vi "Load Custom Test Config Data.vi"(8 "Error In":errorcluster, 9 "Challenge Config Directory":path, 10 "Challenge Config":T1, 11 "Config File Handle":T2) -> (0 "Error Out":errorcluster, 1 "Challenge Config Directory":path, 2 "Challenge Config":T1, 3 "Config File Handle":T2)   [LabVIEW 2013, in "VIChallenge.lvlib"]
doc: "Load custom tests by reading from the challenge config file."
uses:
  VIChallenge.lvlib
  <vilib>/Utility/config.llb/Config Data RefNum.ctl
  Type Defs/Challenge.ctl
  <vilib>/Utility/config.llb/Read Key (Boolean).vi
  <vilib>/Utility/config.llb/NI_LVConfig.lvlib
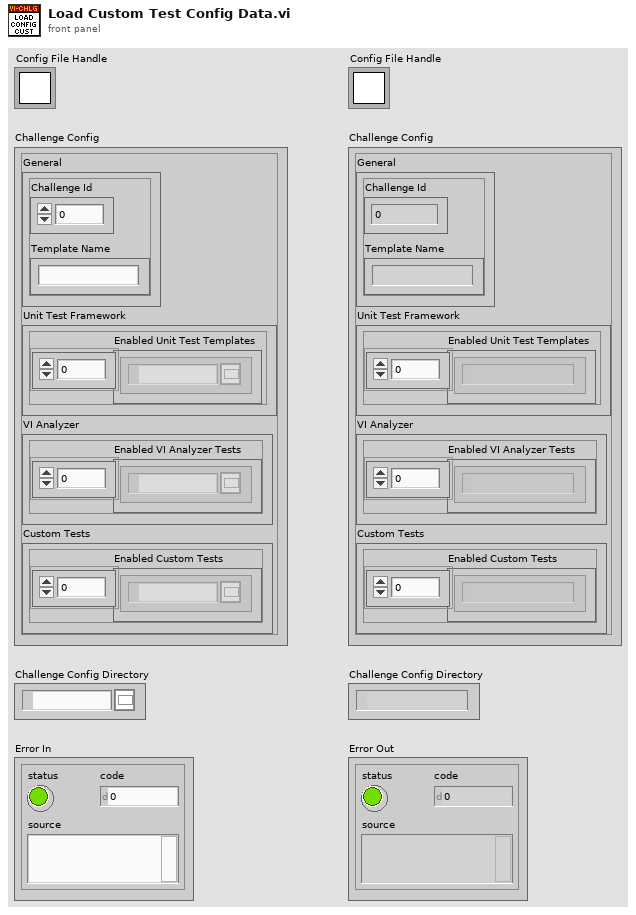
[diagram p1: front panel]
types:
  T1 = typedef "VIChallenge.lvlib/Challenge.ctl" = cluster{"General":cluster{"Challenge Id":i32, "Template Name":string}, "Unit Test Framework":cluster{"Enabled Unit Test Templates":path[]}, "VI Analyzer":cluster{"Enabled VI Analyzer Tests":path[]}, "Custom Tests":cluster{"Enabled Custom Tests":path[]}}
  T2 = typedef "NI_LVConfig.lvlib/Config Data RefNum.ctl" = refnum<k1>
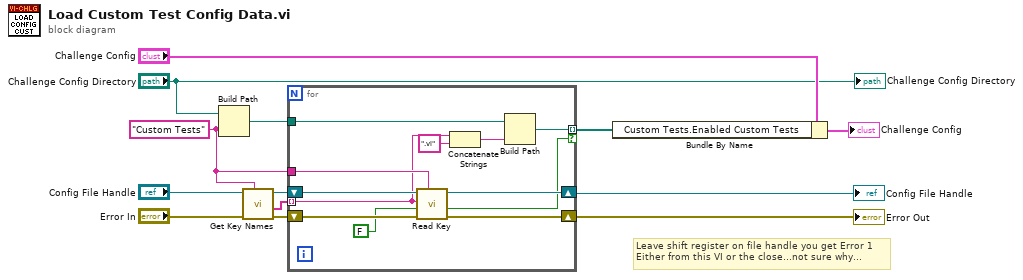
[diagram p0: block diagram]
diagram:
  w1 = "Custom Tests" ("name or relative path")
  # "Leave shift register on file handle you get Error 1\nEither from this VI or the close...not sure why..."
  n1 = Build Path(base path="Challenge Config Directory", name or relative path=w1) -> (appended path=w2:path)
  n2 = call <vilib>:"Get Key Names.vi"("section"=w1, "error in (no error)"="Error In", "refnum"="Config File Handle") -> ("error out"=w9:errorcluster, "key names"=w11:string[], "refnum out"=w10:T2)  [unwired: 5 in, 1 out]
  n3 = for {
    tunnel: w11 -> [w16] mode=indexing
    tunnel: w1 -> [w22]
    shift-right: [w20] -> w13
    shift-left: w9 -> [w25]
    tunnel: [w19] -> w4 mode=indexing if=w18
    tunnel: w2 -> [w17]
    shift-right: [w21] -> w12
    shift-left: w10 -> [w24]
    n4 = call-poly <vilib>:"Read Key.vi"("section"=w22, "error in (no error)"=w25, "default value"=FALSE, "key"=w16, "refnum"=w24) -> ("error out"=w20:errorcluster, "value"=w18:bool, "refnum out"=w21:T2)  [unwired: 3 in, 1 out]
    n5 = Concatenate Strings(w16, ".vi" ("string")) -> (w15:string)
    n6 = Build Path(base path=w17, name or relative path=w15) -> (appended path=w19:path)
  }
  "Error Out" <- w13
  "Config File Handle" <- w12
  n7 = Bundle By Name(cluster="Challenge Config", "Custom Tests.Enabled Custom Tests"=w4) -> (→"Challenge Config":T1)
  "Challenge Config Directory" <- "Challenge Config Directory"
